vi "Island Control.vi"(8 "error in (no error)":errorcluster, 10 "IED Name":string, 11 "SCADA in":refnum<class "SCADA.lvclass">) -> (0 "error out":errorcluster, 3 "SCADA out":refnum<class "SCADA.lvclass">)   [LabVIEW 2015, in "SCADA Core.lvlib" / "SCADA.lvclass"]
uses:
  SCADA.lvclass
  Controls/Queue Selector.ctl
  <vilib>/Utility/error.llb/DialogType.ctl
  SCADA Abstract Messages/Device Action Status Msg/Device Action Status.ctl
  <vilib>/ActorFramework/Actor/Actor.lvclass/Actor.ctl
  <vilib>/ActorFramework/Message Enqueuer/Message Enqueuer.lvclass/Message Enqueuer.ctl
  SCADA Response Messages/Return Island Control Status Msg/Return Island Control Status Msg.lvclass/Return Island Control Status Msg.ctl
  SCADA.lvclass/SCADA.ctl
  <vilib>/ActorFramework/Message Enqueuer/Init from Existing Queue.vi
  <vilib>/ActorFramework/Message Enqueuer/Enqueue.vi
  <vilib>/ActorFramework/Message Priority Queue/Priority Enqueue.vi
  <vilib>/ActorFramework/Message Enqueuer/Message Enqueuer.lvclass
  SCADA Response Messages/Return Island Control Status Msg/Return Island Control Status Msg.lvclass
  IED Actor/IED Messages/Set Device as Islanding Control Msg/Set Device as Islanding Control Msg.lvclass
  SCADA Abstract Messages/Device Action Status Msg/Device Action Status Msg.lvclass
  <vilib>/ActorFramework/Actor/Actor.lvclass
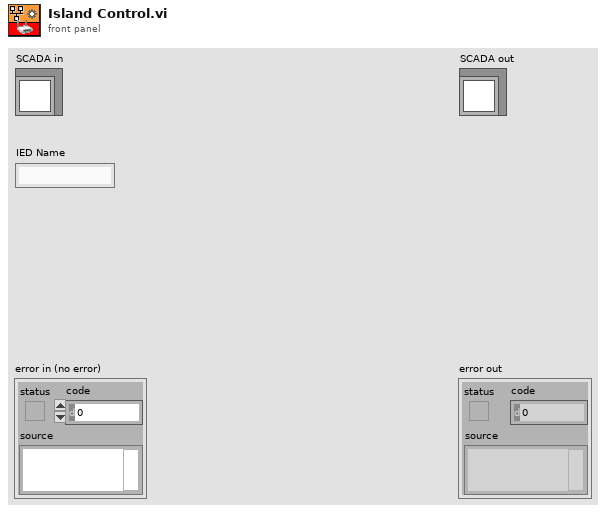
[diagram p1: front panel]
types:
  T1 = typedef "SCADA Core.lvlib/SCADA.lvclass/Queue Selector.ctl" = enum16{"IEDs", "PV", "Generators", "Wind", "Storage", "Relays"}
  T2 = typedef "SCADA Core.lvlib/Device Action Status Msg.lvclass/Device Action Status.ctl" = enum16{"Success", "Failure"}
  T3 = typedef "DialogType.ctl" = u16
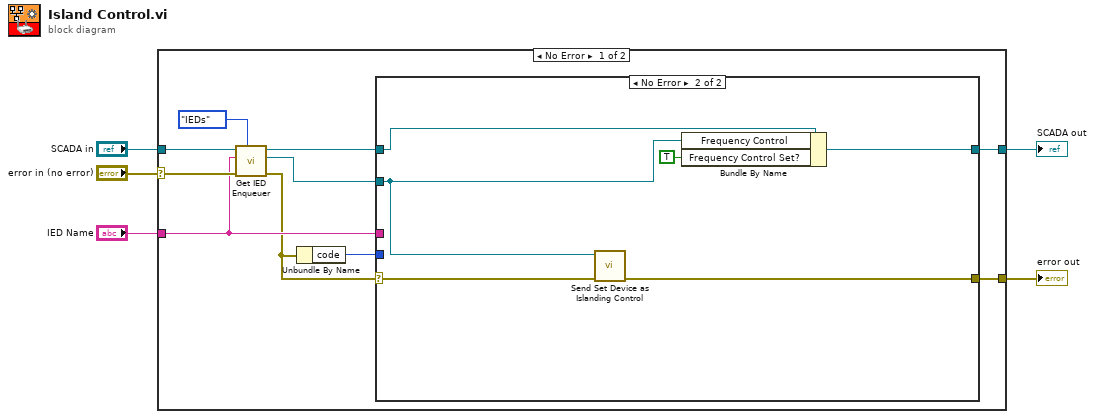
[diagram p0: block diagram]
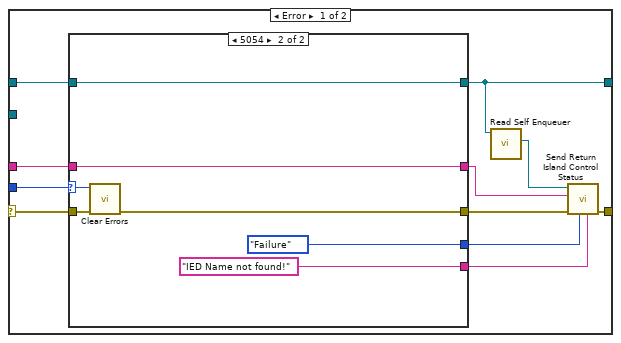
[diagram p2: hidden frame]
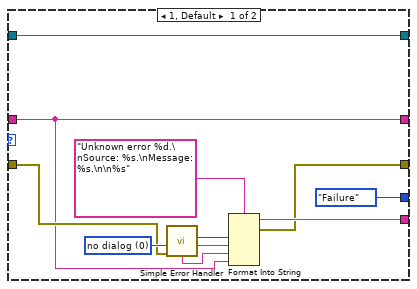
[diagram p3: hidden frame]
diagram:
  n1 = case shown="No Error" "error in (no error)" {
    selector: "error in (no error)" -> [w13 w52]
    tunnel: [w6 w52] -> w4
    tunnel: [w8 w51] -> w2
    tunnel: "SCADA in" -> [w14 w51]
    tunnel: "IED Name" -> [w11 _]
    frame No Error {
      n2 = call "Get IED Enqueuer.vi"("Queue (IEDs)"=Queue_Selector."IEDs" ("Queue"), "error in (no error)"=w13, "IED Name"=w11, "SCADA in"=w14) -> ("error out"=w7:errorcluster, "IED Enqueuer"=w9:refnum<class "Message Enqueuer.lvclass">, "SCADA out"=w10:refnum<class "SCADA.lvclass">)  [unwired: 5 in]
      n3 = Unbundle By Name(w7) -> ("code"=w12:i32)
      n4 = case shown="No Error" w7 {
        selector: w7 -> [w23 w47]
        tunnel: w12 -> [w26 _]
        tunnel: w11 -> [w25 _]
        tunnel: w10 -> [w24 w50]
        tunnel: w9 -> [_ w48]
        tunnel: [w16 w49] -> w8
        tunnel: [w17 w46] -> w6
        frame Error {
          n5 = case shown="5054" w26 {
            selector: w26 -> [_ w43]
            tunnel: w23 -> [w32 w44]
            tunnel: [w29 w42] -> w20
            tunnel: [Device_Action_Status."Failure" ("Status") Device_Action_Status."Failure" ("Status")] -> w19
            tunnel: [w31 "IED Name not found!" ("error string")] -> w18
            tunnel: [w28 w38] -> w21
            tunnel: w25 -> [w28 w38]
            tunnel: w24 -> [w27 w39]
            tunnel: [w27 w39] -> w16
            frame 1, Default {
              w33 = T3 0 items=["no dialog", "OK message", "continue or stop message", "OK message + warnings", "continue/stop + warnings"] ("type of dialog (OK msg:1)")
              n6 = call <vilib>:"Simple Error Handler.vi"("type of dialog (OK msg:1)"=w33, "error in (no error)"=w32) -> ("code out"=w35:i32, "source out"=w36:string, "message"=w37:string)  [unwired: 3 in, 2 out]
              n7 = Format Into String(format string="Unknown error %d.\nSource: %s.\nMessage: %s.\n\n%s" ("Error String"), w35, w36, w37, w28) -> (resulting string=w31:string, error out=w29:errorcluster)  [unwired: 2 in]
            }
            frame 5054 {
              n8 = call <vilib>:"Clear Errors.vi"("error in (no error)"=w44, "specific error code to clear (0: all)"=w43) -> ("error out"=w42:errorcluster)  [unwired: 4 in, 1 out]
            }
          }
          n9 = call <vilib>:"Read Self Enqueuer.vi"("Actor"=w16) -> ("Self Enqueuer"=w22:refnum<class "Message Enqueuer.lvclass">)  [unwired: 10 in]
          n10 = call "Send Return Island Control Status.vi"("error string"=w18, "Status"=w19, "error in (no error)"=w20, "IED Name"=w21, "Message Enqueuer"=w22) -> ("error out"=w17:errorcluster)  [unwired: 5 in, 1 out]
        }
        frame No Error {
          n11 = call "Send Set Device as Islanding Control.vi"("error in (no error)"=w47, "Message Enqueuer"=w48) -> ("error out"=w46:errorcluster)  [unwired: 8 in, 1 out]
          n12 = Bundle By Name(cluster=w50, "Frequency Control"=w48, "Frequency Control Set?"=TRUE) -> (w49:refnum<class "SCADA.lvclass">)
        }
      }
    }
    frame Error {
    }
  }
  "error out" <- w4
  "SCADA out" <- w2
